vi "DSF.Engine.Interface.Plugin.Destroy.vi"(8 "error in (no error)":errorcluster, 11 "Plugin Interface in":refnum<class "DSF.Engine.Interface.Plugin.lvclass">) -> (0 "error out":errorcluster)   [LabVIEW 2016, in "DSF.Engine.lvlib" / "DSF.Engine.Interface.Plugin.lvclass"]
uses:
  DSF.Engine.Interface.Plugin.lvclass
  C:/Git/Sourcetree/DSF/Source/Engine/Classes/Interface/DSF.Engine.Interface.lvclass
  DSF.Engine.Interface.lvclass
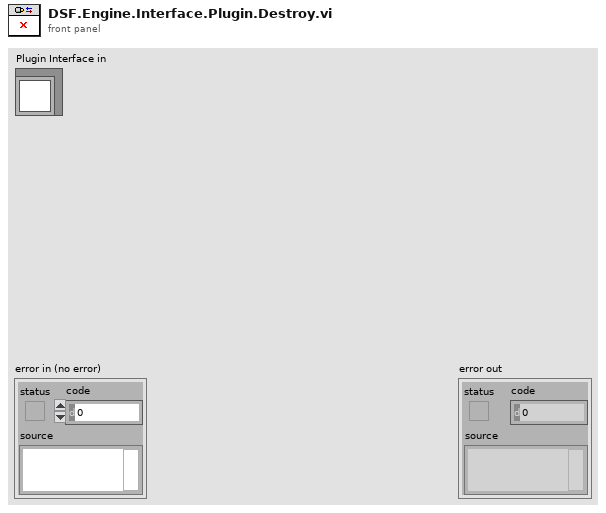
[diagram p1: front panel]
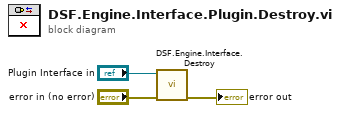
[diagram p0: block diagram]
diagram:
  n1 = call "DSF.Engine.Interface.Destroy.vi"("error in (no error)"="error in (no error)", "Interface in"="Plugin Interface in") -> ("error out"=→"error out":errorcluster)  [unwired: 8 in, 1 out]
